vi "Time_elapsed.vi"(4 "End of previous average in":dbl, 7 "Averaging time (mins)":dbl format="%.2f") -> (0 "End of previous average out":dbl, 1 "End of period":dbl, 2 "Start of period":dbl, 3 "Time elapsed ?":bool)   [LabVIEW 2010]
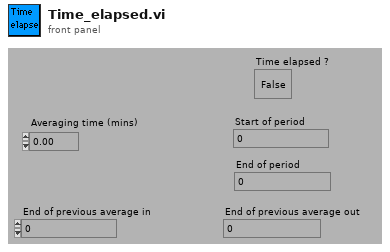
[diagram p1: front panel]
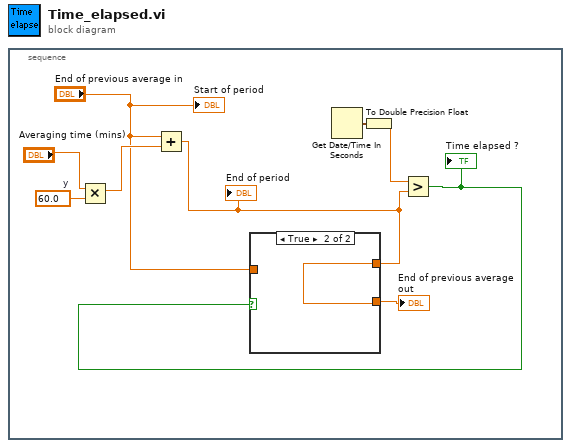
[diagram p0: block diagram]
diagram:
  n1 = stacked-sequence {
    frame #0 {
      w9 = 60.0  # y
      n2 = Multiply(x="Averaging time (mins)", y=w9) -> (x*y=w7:dbl)
      n3 = Add(x="End of previous average in", y=w7) -> (x+y=w3:dbl)
      "End of period" <- w3
      n4 = Get Date/Time In Seconds() -> (seconds since 1Jan1904=w1:timestamp)
      n5 = To Double Precision Float(number=w1) -> (double precision float=w6:dbl)
      n6 = Greater?(x=w6, y=w3) -> (0:w2:bool)
      "Time elapsed ?" <- w2
      n7 = case shown="True" w2 {
        tunnel: [w10 w11] -> w5
        tunnel: "End of previous average in" -> [w10 _]
        tunnel: w3 -> [_ w11]
        frame False {
        }
        frame True {
        }
      }
      "End of previous average out" <- w5
      "Start of period" <- "End of previous average in"
    }
  }
